vi "Transport.vi"(4 "Queue of Error":refnum<queue>, 6 "Queue of Self Attributes":refnum<queue>, 7 "Actor in":refnum<class "Actor.lvclass">, 10 "Attributes":refnum<class "Attributes.lvclass">) -> (0 "Error out":errorcluster, 5 "Actor out":refnum<class "Actor.lvclass">)   [LabVIEW 2025, in "jettl.lvlib" / "Transport.lvlib" / "Event.lvlib"]
uses:
  Event.lvlib
  Attributes/Attributes/Attributes.lvclass
  Actor/Actor.lvclass
  jettl.lvlib
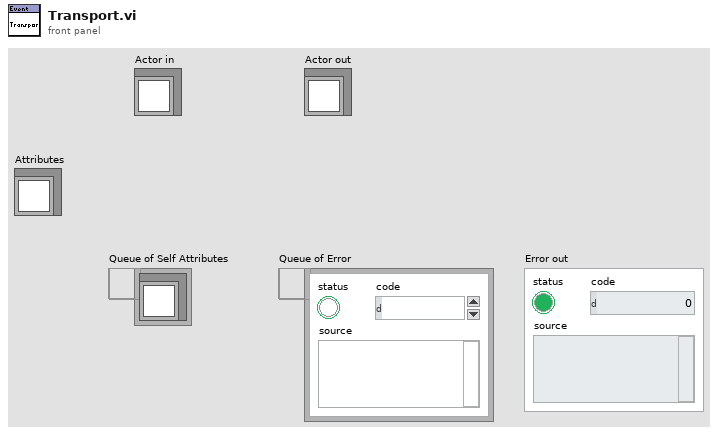
[diagram p1: front panel]
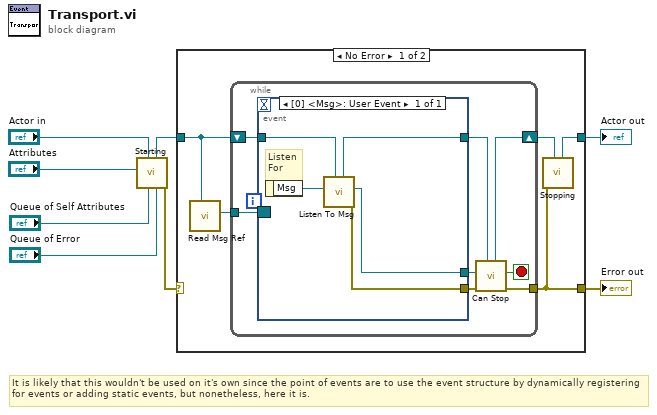
[diagram p0: block diagram]
diagram:
  # "It is likely that this wouldn't be used on it's own since the point of events are to use the event structure by dynamically registering for events or adding static events, but nonetheless, here it is."
  n1 = call "Starting.vi"("Queue of Error"="Queue of Error", "Queue of Self Attributes"="Queue of Self Attributes", "Actor in"="Actor in", "Attributes"="Attributes") -> ("Error out"=w6:errorcluster, "Actor out"=w7:refnum<class "Actor.lvclass">)  [unwired: 6 in]
  n2 = case shown="No Error" w6 {
    selector: w6 -> [_ w27]
    tunnel: [w11 w28] -> w2
    tunnel: w7 -> [w10 w28]
    tunnel: [w13 w27] -> w8
    frame No Error {
      n3 = call "Read Msg Ref.vi"("Actor"=w10) -> ("Msg Ref"=w9:refnum<event-registration>)  [unwired: 10 in]
      n4 = while {
        shift-right: [w17] -> w12
        shift-left: w10 -> [w20]
        tunnel: w9 -> [w21]
        tunnel: [w18] -> w13
        stop <- w16 stop-if-true
        n5 = event shown="[0] <Msg>: User Event" {
          selector: w21 -> [_]
          dyn-events: _ -> [_]
          timeout: _ -> [_]
          tunnel: w20 -> [w26]
          tunnel: [w24] -> w15
          tunnel: [w23] -> w19
          tunnel: [w22] -> w14
          event User Event {
            # "Listen\nFor"
            n6 = event-data() -> ("Msg"=w25:refnum<class "Msg.lvclass">)  [unwired: 1 in]
            n7 = call "Listen To Msg.vi"("Actor in"=w26, "Msg"=w25) -> ("Error out"=w23:errorcluster, "Msg Output"=w22:refnum<class "Msg Output.lvclass">, "Actor out"=w24:refnum<class "Actor.lvclass">)  [unwired: 7 in]
          }
        }
        n8 = call "Can Stop.vi"("Actor in"=w15, "Error in"=w19, "Msg Output"=w14) -> ("Error out"=w18:errorcluster, "Stop"=w16:bool, "Actor out"=w17:refnum<class "Actor.lvclass">)  [unwired: 6 in]
      }
      n9 = call "Stopping.vi"("Actor in"=w12, "Error in"=w13) -> ("Actor out"=w11:refnum<class "Actor.lvclass">)  [unwired: 9 in]
    }
    frame Error {
    }
  }
  "Error out" <- w8
  "Actor out" <- w2
